vi "Graph.vi"() -> ()   [LabVIEW 2019]
panel:
  in  "Array":dbl[](array[numeric])
  out "Waveform Graph":dbl[](graph)
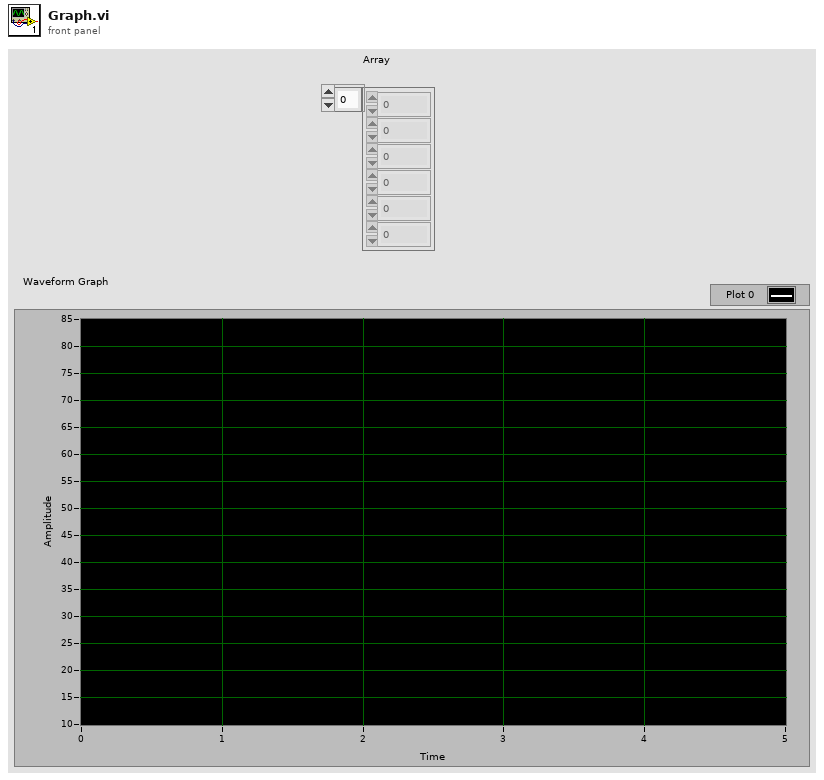
[diagram p1: front panel]
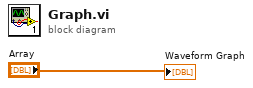
[diagram p0: block diagram]
diagram:
  "Waveform Graph" <- "Array"
